vi "AI-loop-unitest.vi"(8 "错误输入（无错误）":errorcluster, 11 "Status":T1 {"Setting"."X Pos." scale=-5.0..5.0; "Setting"."Y Pos." scale=-5.0..5.0}) -> (0 "Error out":errorcluster caption="错误输入（无错误）")   [LabVIEW 2013]
uses:
  init/init-status.ctl
  init/Setting.ctl
  event-package.ctl
  Event1.ctl
  data-package.ctl
  Event.ctl
  <vilib>/DAQmx/read.llb/DAQmx Read (Analog 1D DBL 1Chan NSamp).vi
  <vilib>/DAQmx/create/channels.llb/DAQmx Create Channel (AI-Voltage-Basic).vi
  <vilib>/DAQmx/configure/timing.llb/DAQmx Timing (Sample Clock).vi
  <vilib>/DAQmx/configure/trigger.llb/DAQmx Start Trigger (Digital Edge).vi
  <vilib>/DAQmx/miscellaneous.llb/DAQmx Fill In Error Info.vi
panel:
  out "line #":i32
  out "波形图":dbl[](graph)
  out "frame #":i32
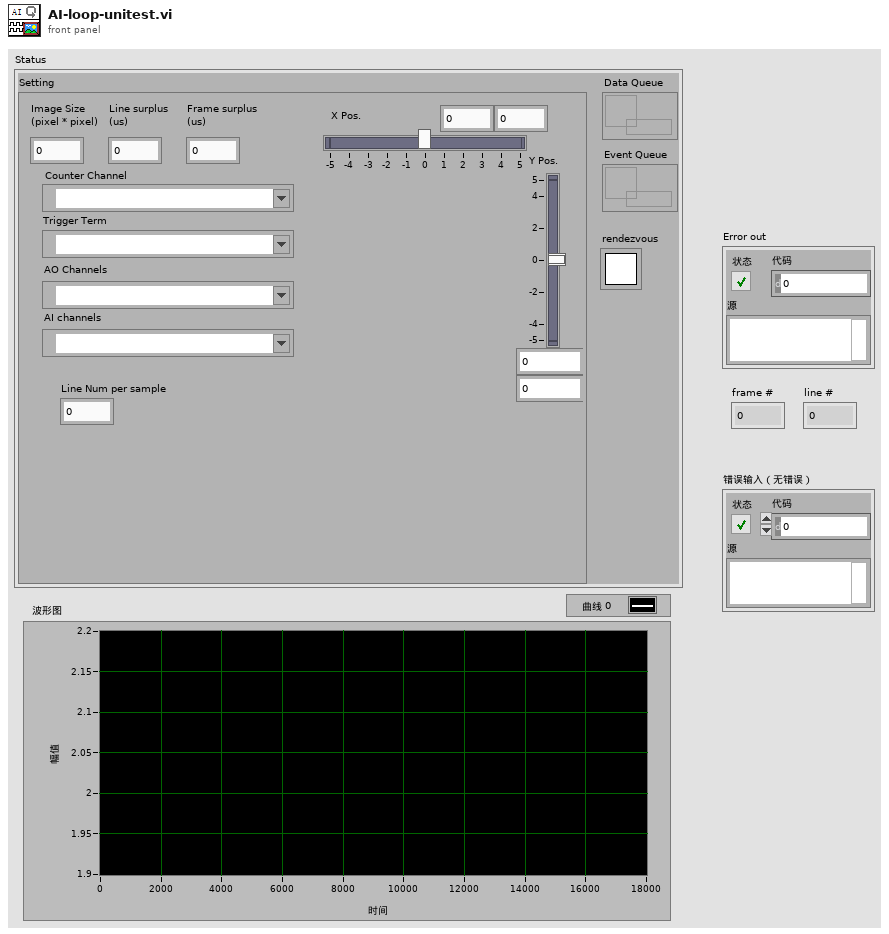
[diagram p1: front panel]
types:
  T1 = typedef "init-status.ctl" = cluster{"Setting":T2, "Event Queue":refnum<queue>, "Data Queue":refnum<queue>, "rendezvous":T3}
  T2 = typedef "Setting.ctl" = cluster{"Image Size\n(pixel * pixel)":i32, "Counter Channel":tag, "Trigger Term":tag, "AO Channels":tag, "Y Pos.":cluster{dbl, dbl}, "X Pos.":cluster{dbl, dbl}, "Line surplus\n(us)":i32, "Frame surplus\n(us)":i32, "AI channels":tag, "Line Num per sample":i32}
  T3 = typedef "Rendezvous RefNum" = refnum<k1>
  T4 = typedef "data-package.ctl" = cluster{"Event":T5, "Data":dbl[], "line #":i32}
  T5 = typedef "Event.ctl" = u16
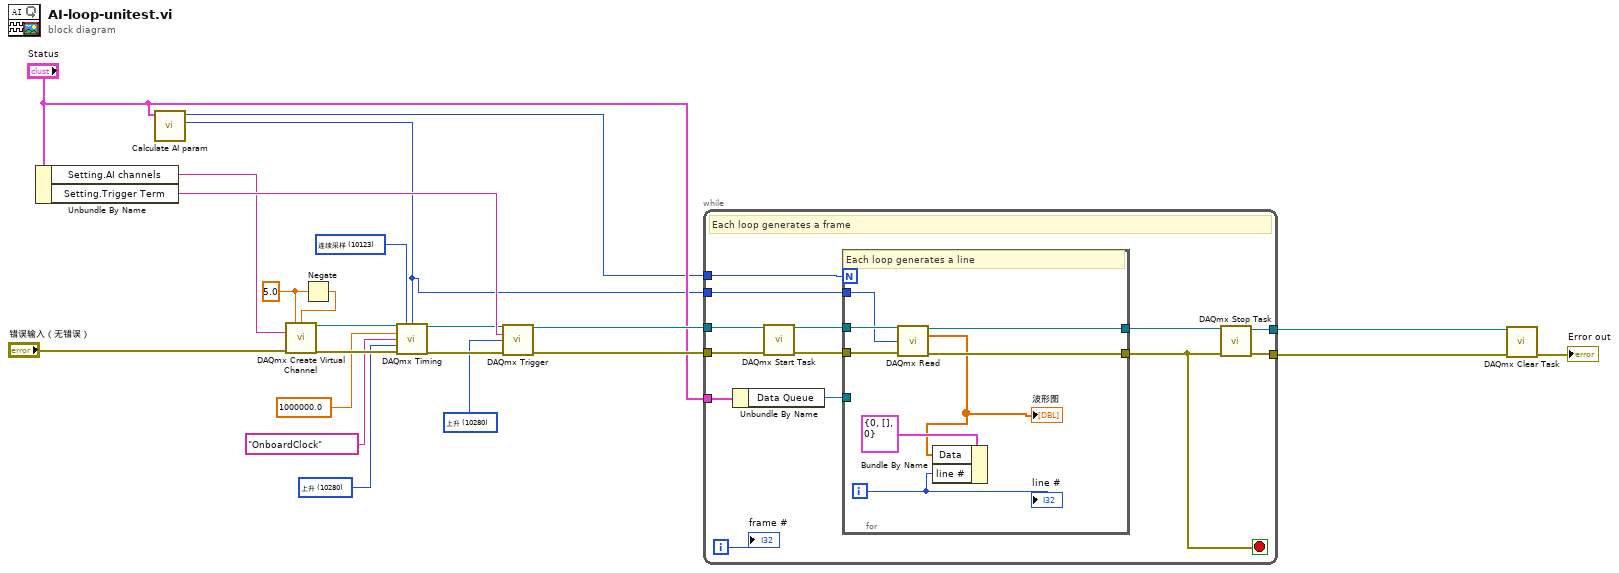
[diagram p0: block diagram]
diagram:
  w9 = 10280 items=["上升"=10280, "下降"=10171] ("edge")
  w12 = 10123 items=["有限采样"=10178, "连续采样"=10123, "硬件定时单点"=12522] ("sample mode")
  w13 = 10280 items=["上升"=10280, "下降"=10171] ("active edge")
  w19 = 5.0
  n1 = Unbundle By Name("Status") -> ("Setting.AI channels"=w20:tag, "Setting.Trigger Term"=w21:tag)
  n2 = call "Calculate AI param.vi"("Status"="Status") -> ("# samples per channel"=w2:i32, "# channels per frame"=w1:i32)  [unwired: 9 in]
  n3 = Negate(x=w19) -> (-x=w18:dbl)
  n4 = call-poly <vilib>:"DAQmx Create Virtual Channel.vi"("maximum value"=w19, "minimum value"=w18, "physical channels"=w20, "error in"="错误输入（无错误）") -> ("task out"=w17:refnum<k21>, "error out"=w16:errorcluster)  [unwired: 10 in]
  n5 = call-poly <vilib>:"DAQmx Timing.vi"("task/channels in"=w17, "sample mode"=w12, "samples per channel"=w2, "rate"=1000000.0, "source"=tag "OnboardClock", "active edge"=w13, "error in"=w16) -> ("task out"=w11:refnum<k21>, "error out"=w10:errorcluster)  [unwired: 7 in]
  n6 = call-poly <vilib>:"DAQmx Trigger.vi"("task/channels in"=w11, "source"=w21, "edge"=w9, "error in"=w10) -> ("task out"=w7:refnum<k21>, "error out"=w6:errorcluster)  [unwired: 10 in]
  n7 = while {
    tunnel: w7 -> [w31]
    tunnel: w6 -> [w30]
    tunnel: [w26] -> w4
    tunnel: [w25] -> w5
    tunnel: "Status" -> [w35]
    tunnel: w2 -> [w32]
    tunnel: w1 -> [w23]
    i -> [w33]
    stop <- w27 stop-if-true
    # "Each loop generates a frame"
    n8 = Unbundle By Name(w35) -> ("Data Queue"=w34:refnum<queue>)
    n9 = call <vilib>:"DAQmx Start Task.vi"("task/channels in"=w31, "error in"=w30) -> ("task out"=w28:refnum<k21>, "error out"=w29:errorcluster)  [unwired: 12 in]
    n10 = for {
      N: w23 -> [_]
      tunnel: w28 -> [w43]
      tunnel: w29 -> [w42]
      tunnel: [w41] -> w27
      tunnel: [w40] -> w24
      tunnel: w34 -> [_]
      tunnel: w32 -> [w37]
      i -> [w38]
      # "Each loop generates a line"
      n11 = call-poly <vilib>:"DAQmx Read.vi"("task/channels in"=w43, "number of samples per channel"=w37, "error in"=w42) -> ("task out"=w40:refnum<k21>, "data"=w36:dbl[], "error out"=w41:errorcluster)  [unwired: 10 in]
      "波形图" <- w36
      n12 = Bundle By Name(cluster=T4 {"Event"=0, "Data"=[], "line #"=0} ("Data Package"), "Data"=w36, "line #"=w38) -> ()  [unwired: 1 out]
      "line #" <- w38
    }
    n13 = call <vilib>:"DAQmx Stop Task.vi"("task/channels in"=w24, "error in"=w27) -> ("task out"=w25:refnum<k21>, "error out"=w26:errorcluster)  [unwired: 12 in]
    "frame #" <- w33
  }
  n14 = call <vilib>:"DAQmx Clear Task.vi"("task in"=w5, "error in"=w4) -> ("error out"=→"Error out":errorcluster)  [unwired: 13 in]
